vi "Num_Str_Zusammen.vi"(1 "Color Box":u32(colorbox), 2 "string":string, 3 "number":dbl) -> (0 "Array":u32[][](array[numeric]))   [LabVIEW 2021]
panel:
  out "size(s)":i32[](array[numeric])
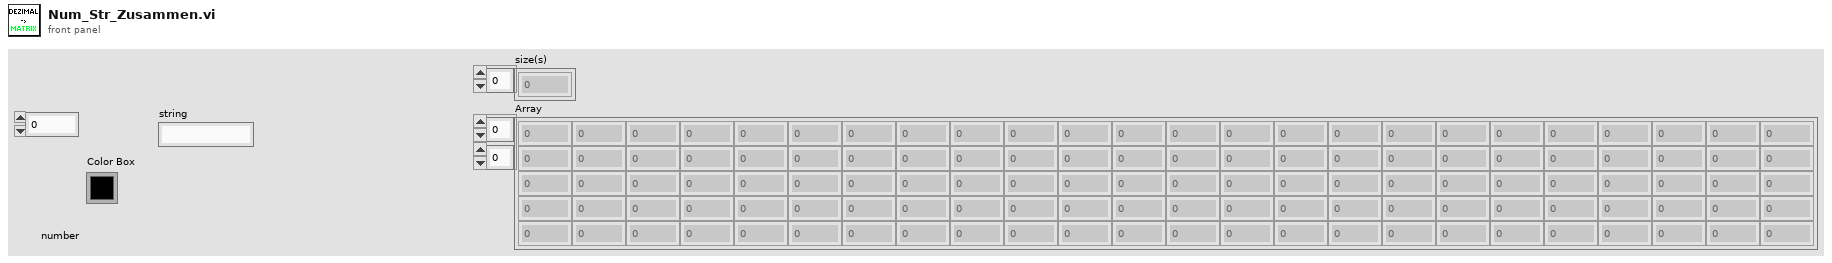
[diagram p1: front panel]
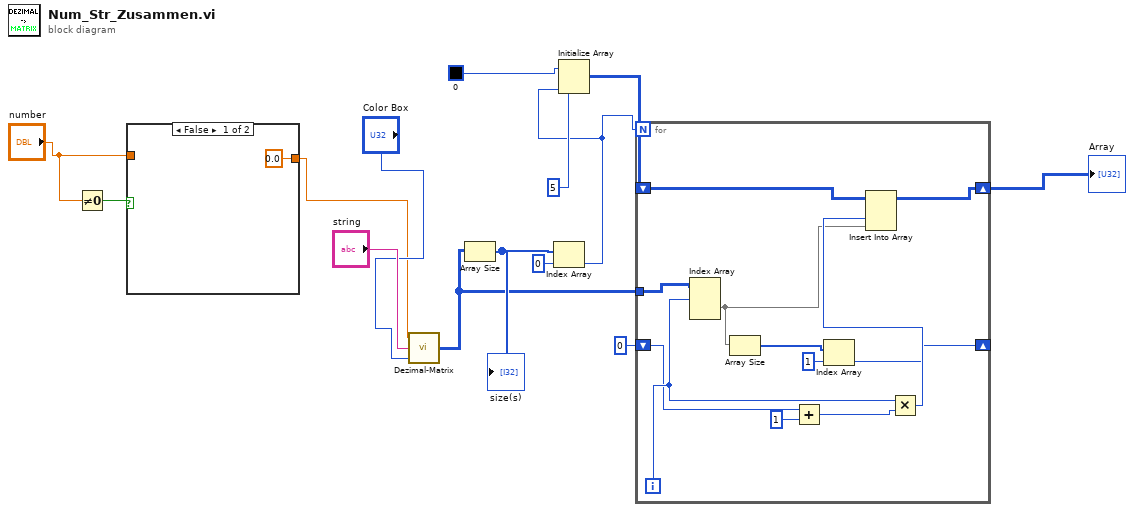
[diagram p0: block diagram]
diagram:
  n1 = Not Equal To 0?(x="number") -> (x != 0?=w2:bool)
  n2 = case shown="False" w2 {
    tunnel: "number" -> [_ w16]
    tunnel: [0.0 ("number") w16] -> w3
    frame False {
    }
    frame True {
    }
  }
  n3 = call "Dezimal-Matrix.vi"("Color Box"="Color Box", "string"="string", "number"=w3) -> ("output array"=w10:u32[][][])
  n4 = Array Size(array=w10) -> (size(s)=w13:i32[])
  "size(s)" <- w13
  n5 = Index Array(array=w13, index=0) -> (element=w4:i32)
  n6 = Initialize Array(u32 0 ("Color Box"), 5 ("dimension size"), w4) -> (w7:u32[][])
  n7 = for {
    N: w4 -> [_]
    tunnel: w10 -> [w28]
    shift-right: [w27] -> w9
    shift-left: w7 -> [w26]
    shift-right: [w20] -> _
    shift-left: 0 -> [w18]
    i -> [w25]
    n8 = Index Array(array=w28, index (dim 0)=w25) -> (element=w23:u32[][])  [unwired: 2 in]
    n9 = Array Size(array=w23) -> (size(s)=w22:i32[])
    n10 = Add(x=w18, y=1) -> (x+y=w19:i32)
    n11 = Index Array(array=w22, index=1) -> (element=w20:i32)
    n12 = Multiply(x=w25, y=w19) -> (x*y=w24:i32)
    n13 = Insert Into Array(array=w26, index (col)=w24, new element=w23) -> (w27:u32[][])  [unwired: 1 in]
  }
  "Array" <- w9
